vi "Scan.vi"(8 "error in":errorcluster, 11 "variant in":variant) -> (0 "error out":errorcluster, 3 "variant out":variant, 4 "Scanning":bool)   [LabVIEW 2013]
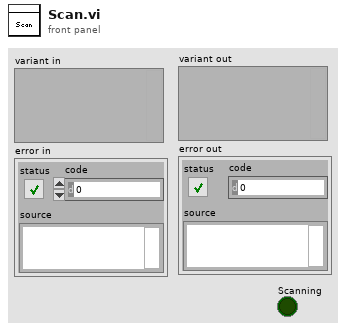
[diagram p1: front panel]
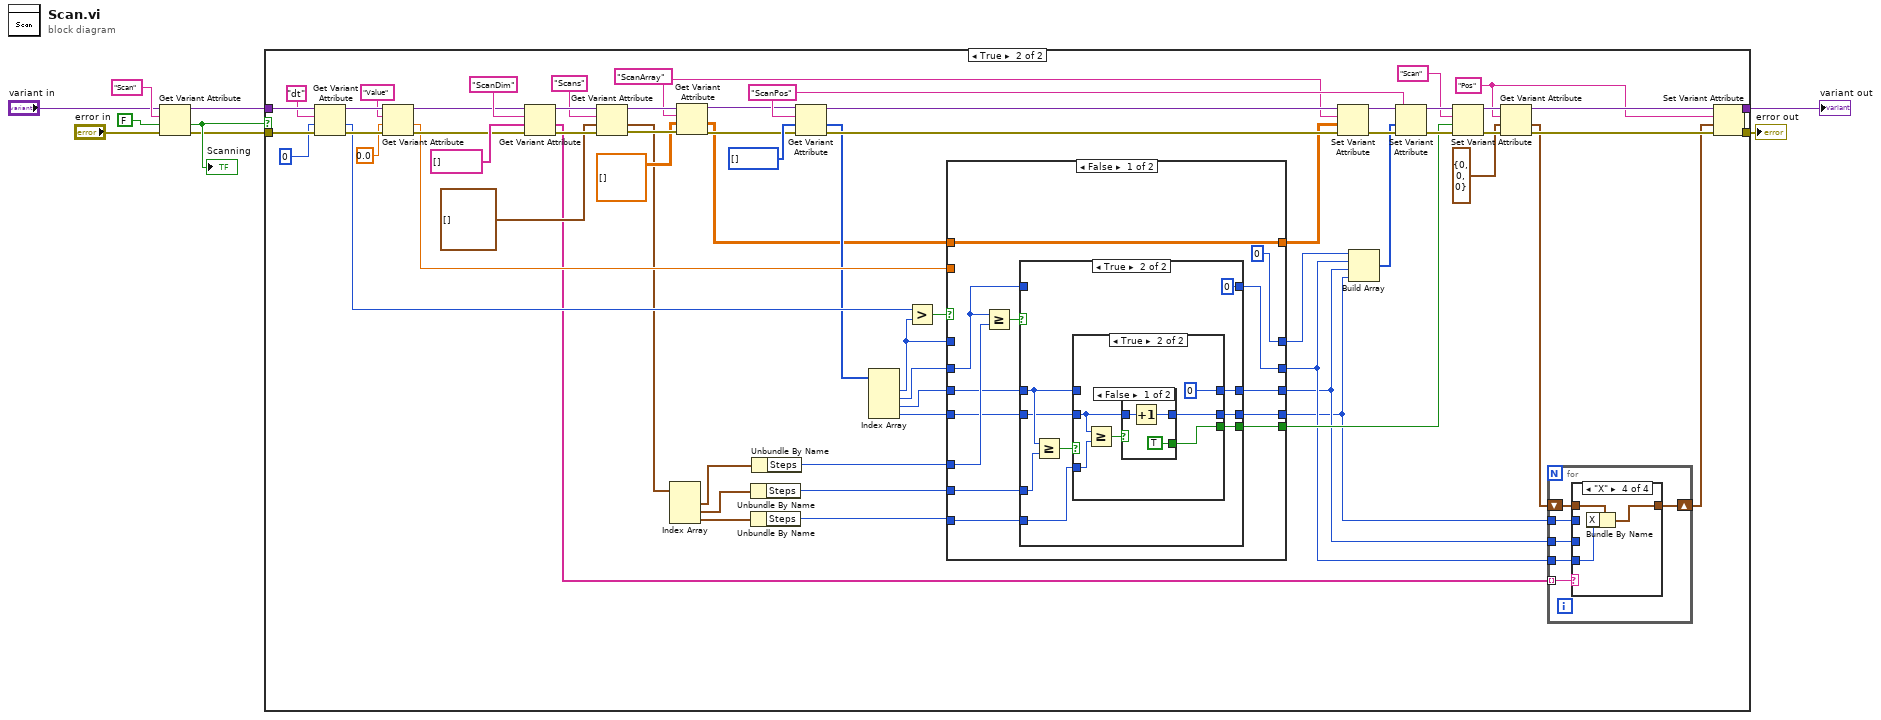
[diagram p0: block diagram]
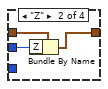
[diagram p4: hidden frame]
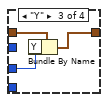
[diagram p5: hidden frame]
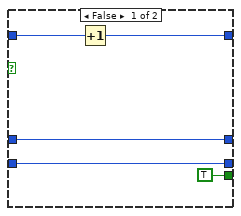
[diagram p6: hidden frame]
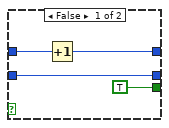
[diagram p7: hidden frame]
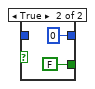
[diagram p8: hidden frame]
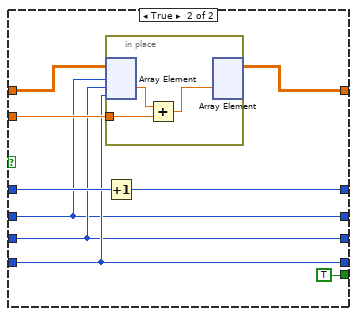
[diagram p9: hidden frame]
diagram:
  n1 = Get Variant Attribute(Variant="variant in", name="Scan", default value (empty Variant)=FALSE, error in="error in") -> (duplicate Variant=w7:variant, value=w9:bool, error out=w8:errorcluster)  [unwired: 1 out]
  "Scanning" <- w9
  n2 = case shown="True" w9 {
    tunnel: [w11 w26] -> w2
    tunnel: w7 -> [w11 w71]
    tunnel: [w10 w25] -> w1
    tunnel: w8 -> [w10 w70]
    frame False {
    }
    frame True {
      w19 = "Pos" ("name")
      w43 = "ScanArray" ("name")
      w72 = "ScanPos" ("name")
      n3 = Get Variant Attribute(Variant=w71, name="dt", default value (empty Variant)=0, error in=w70) -> (duplicate Variant=w64:variant, value=w58:i32, error out=w61:errorcluster)  [unwired: 1 out]
      n4 = Get Variant Attribute(Variant=w64, name="Value", default value (empty Variant)=0.0, error in=w61) -> (duplicate Variant=w63:variant, value=w48:dbl, error out=w62:errorcluster)  [unwired: 1 out]
      n5 = Get Variant Attribute(Variant=w63, name="ScanDim", default value (empty Variant)=string[] [], error in=w62) -> (duplicate Variant=w76:variant, value=w18:string[], error out=w75:errorcluster)  [unwired: 1 out]
      n6 = Get Variant Attribute(Variant=w76, name="Scans", default value (empty Variant)=cluster{"Start":dbl, "Stop":dbl, "Steps":u32}[] [], error in=w75) -> (duplicate Variant=w56:variant, value=w41:cluster{"Start":dbl, "Stop":dbl, "Steps":u32}[], error out=w53:errorcluster)  [unwired: 1 out]
      n7 = Index Array(array=w41) -> (element #1=w40:cluster{"Start":dbl, "Stop":dbl, "Steps":u32}, element #2=w39:cluster{"Start":dbl, "Stop":dbl, "Steps":u32}, element #3=w38:cluster{"Start":dbl, "Stop":dbl, "Steps":u32})  [unwired: 3 in]
      n8 = Get Variant Attribute(Variant=w56, name=w43, default value (empty Variant)=dbl[][][] [] ("initialized array"), error in=w53) -> (duplicate Variant=w55:variant, value=w24:dbl[][][], error out=w54:errorcluster)  [unwired: 1 out]
      n9 = Unbundle By Name(w39) -> ("Steps"=w35:u32)
      n10 = Unbundle By Name(w38) -> ("Steps"=w34:u32)
      n11 = Unbundle By Name(w40) -> ("Steps"=w37:u32)
      n12 = Get Variant Attribute(Variant=w55, name=w72, default value (empty Variant)=i32[] [], error in=w54) -> (duplicate Variant=w47:variant, value=w36:i32[], error out=w46:errorcluster)  [unwired: 1 out]
      n13 = Index Array(array=w36) -> (element #1=w33:i32, element #2=w51:i32, element #3=w50:i32, element #4=w49:i32)  [unwired: 4 in]
      n14 = Greater?(x=w58, y=w33) -> (0:w57:bool)
      n15 = case shown="False" w57 {
        tunnel: w24 -> [w105 w141]
        tunnel: w51 -> [w102 w135]
        tunnel: w50 -> [w101 w136]
        tunnel: w49 -> [w100 w137]
        tunnel: w48 -> [_ w139]
        tunnel: [w105 w140] -> w42
        tunnel: w37 -> [w104 _]
        tunnel: w35 -> [w99 _]
        tunnel: w34 -> [w98 _]
        tunnel: [w97 TRUE] -> w27
        tunnel: [w96 w135] -> w17
        tunnel: [w95 w136] -> w16
        tunnel: [w94 w137] -> w15
        tunnel: [0 w142] -> w32
        tunnel: w33 -> [_ w138]
        frame False {
          n16 = Greater Or Equal?(x=w102, y=w104) -> (x >= y?=w103:bool)
          n17 = case shown="True" w103 {
            tunnel: w102 -> [w110 _]
            tunnel: w101 -> [w108 w116]
            tunnel: w100 -> [w107 w114]
            tunnel: [w109 0] -> w96
            tunnel: [w108 w115] -> w95
            tunnel: [w107 w113] -> w94
            tunnel: w99 -> [_ w118]
            tunnel: w98 -> [_ w112]
            tunnel: [TRUE w111] -> w97
            frame False {
              n18 = Increment(x=w110) -> (x+1=w109:i32)
            }
            frame True {
              n19 = Greater Or Equal?(x=w116, y=w118) -> (x >= y?=w117:bool)
              n20 = case shown="True" w117 {
                tunnel: w116 -> [w123 _]
                tunnel: [w122 0] -> w115
                tunnel: w114 -> [w121 w126]
                tunnel: [w121 w125] -> w113
                tunnel: w112 -> [_ w128]
                tunnel: [TRUE w124] -> w111
                frame False {
                  n21 = Increment(x=w123) -> (x+1=w122:i32)
                }
                frame True {
                  n22 = Greater Or Equal?(x=w126, y=w128) -> (x >= y?=w127:bool)
                  n23 = case shown="False" w127 {
                    tunnel: w126 -> [w132 _]
                    tunnel: [w131 0] -> w125
                    tunnel: [TRUE FALSE] -> w124
                    frame False {
                      n24 = Increment(x=w132) -> (x+1=w131:i32)
                    }
                    frame True {
                    }
                  }
                }
              }
            }
          }
        }
        frame True {
          n25 = in-place {
            in-place-border: w139 -> [w144]
            n26 = in-place-array #1(w141, w135, w136, w137) -> (w146:dbl)
            n27 = Add(x=w146, y=w144) -> (x+y=w145:dbl)
            n28 = in-place-array #1(w145) -> (w140:dbl[][][])  [unwired: 3 out]
          }
          n29 = Increment(x=w138) -> (x+1=w142:i32)
        }
      }
      n30 = Set Variant Attribute(Variant=w47, name=w43, value=w42, error in=w46) -> (Variant out=w45:variant, error out=w44:errorcluster)  [unwired: 1 out]
      n31 = Build Array(w32, w17, w16, w15) -> (w31:i32[])
      n32 = Set Variant Attribute(Variant=w45, name=w72, value=w31, error in=w44) -> (Variant out=w30:variant, error out=w29:errorcluster)  [unwired: 1 out]
      n33 = Set Variant Attribute(Variant=w30, name="Scan", value=w27, error in=w29) -> (Variant out=w22:variant, error out=w23:errorcluster)  [unwired: 1 out]
      n34 = Get Variant Attribute(Variant=w22, name=w19, default value (empty Variant)=cluster{"X":u32, "Y":u32, "Z":u32} {"X"=0, "Y"=0, "Z"=0} ("Relative Position"), error in=w23) -> (duplicate Variant=w21:variant, value=w14:cluster{"X":u32, "Y":u32, "Z":u32}, error out=w20:errorcluster)  [unwired: 1 out]
      n35 = for {
        tunnel: w18 -> [w82] mode=indexing
        tunnel: w17 -> [w79]
        tunnel: w16 -> [w80]
        tunnel: w15 -> [w81]
        shift-right: [w77] -> w12
        shift-left: w14 -> [w78]
        n36 = case shown="\"X\"" w82 {
          tunnel: w81 -> [_ w84 _ _]
          tunnel: w80 -> [_ _ w87 _]
          tunnel: w79 -> [_ _ _ w90]
          tunnel: w78 -> [w83 w86 w89 w92]
          tunnel: [w83 w85 w88 w91] -> w77
          frame "none", Default {
          }
          frame "Z" {
            n37 = Bundle By Name(cluster=w86, "Z"=w84) -> (w85:cluster{"X":u32, "Y":u32, "Z":u32})
          }
          frame "Y" {
            n38 = Bundle By Name(cluster=w89, "Y"=w87) -> (w88:cluster{"X":u32, "Y":u32, "Z":u32})
          }
          frame "X" {
            n39 = Bundle By Name(cluster=w92, "X"=w90) -> (w91:cluster{"X":u32, "Y":u32, "Z":u32})
          }
        }
      }
      n40 = Set Variant Attribute(Variant=w21, name=w19, value=w12, error in=w20) -> (Variant out=w26:variant, error out=w25:errorcluster)  [unwired: 1 out]
    }
  }
  "variant out" <- w2
  "error out" <- w1
